vi "TP Buffer Search for Connection (No PGN).vi"(0 "Connecctions":T3[](array[typedef]), 5 "CAN frame":T1 {"payload" format="%x"; "timestamp" format="%<%.7X\n%x>T"; "type" items=["CAN Data"=0, "CAN Remote"=1, "CAN Bus Error"=2, "J1939 Data"=192, "Delay"=224, "Log Trigger"=225, "Start Trigger"=226]; "identifier" format="%x"}, 11 "error in (no error)":errorcluster) -> (4 "Connection Cluster Out":T3, 6 "CAN frame Out":T1 {"payload" format="%x"; "timestamp" format="%<%.7X\n%x>T"; "type" items=["CAN Data"=0, "CAN Remote"=1, "CAN Bus Error"=2, "J1939 Data"=192, "Delay"=224, "Log Trigger"=225, "Start Trigger"=226]; "identifier" format="%x"}, 8 "Found?":bool, 10 "Index":i32, 15 "error out":errorcluster)   [LabVIEW 2013, in "J1939.lvlib"]
uses:
  J1939.lvlib
  TP Buffer Connection Cluster.ctl
  <vilib>/xnet/xnet.llb/XNET Frame CAN.ctl
  <vilib>/xnet/xnet.llb/XNET Frame Type CAN.ctl
  Frame Conversion/Convert CAN Arb ID to J1939 ID.vi
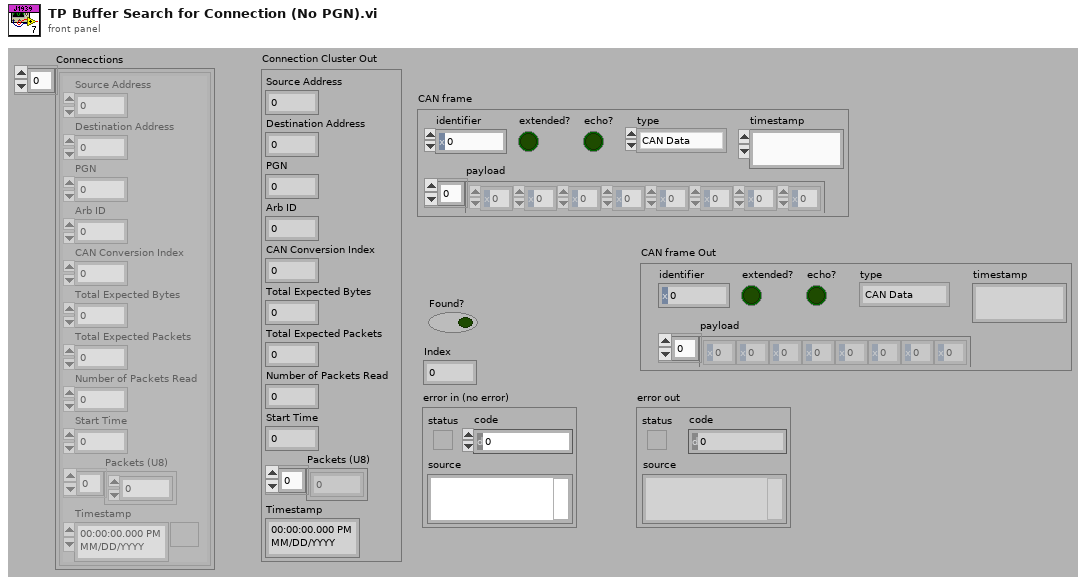
[diagram p1: front panel]
types:
  T1 = typedef "XNET Frame CAN.ctl" = cluster{"timestamp":timestamp, "payload":u8[], "identifier":u32, "type":T2, "extended?":bool, "echo?":bool}
  T2 = typedef "XNET Frame Type CAN.ctl" = u8
  T3 = typedef "J1939.lvlib/TP Buffer Connection Cluster.ctl" = cluster{"Source Address":u8, "Destination Address":u8, "PGN":u32, "Arb ID":u32, "CAN Conversion Index":u32, "Total Expected Bytes":u16, "Total Expected Packets":u8, "Number of Packets Read":u8, "Start Time":u32, "Packets (U8)":u8[], "Timestamp":timestamp}
  T4 = typedef "J1939.lvlib/PGN Fields Cluster.ctl" = cluster{"Reserved Bit":u8, "Data page":u8, "PDU Format":u8, "PDU Specific":u8}
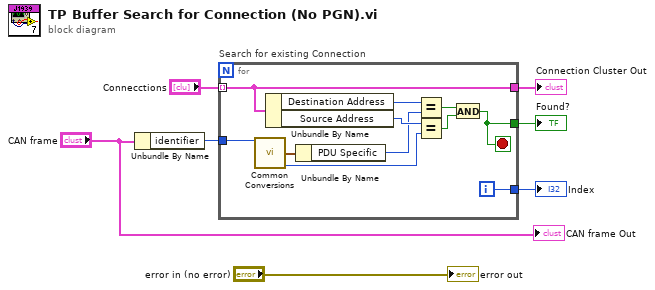
[diagram p0: block diagram]
diagram:
  n1 = Unbundle By Name("CAN frame") -> ("identifier"=w3:u32)
  n2 = for "Search for existing Connection" {
    tunnel: "Connecctions" -> [w9] mode=indexing
    tunnel: w3 -> [w16]
    tunnel: [w10] -> w7
    tunnel: [w9] -> w5
    tunnel: [w8] -> w4
    i -> [w8]
    stop <- w10 stop-if-true
    n3 = call-poly "Common Conversions.vi"("Arb ID"=w16) -> ("PGN Fields"=w17:T4, "Source Address"=w14:u8)  [unwired: 13 out]
    n4 = Unbundle By Name(w9) -> ("Destination Address"=w18:u8, "Source Address"=w15:u8)
    n5 = Unbundle By Name(w17) -> ("PDU Specific"=w13:u8)
    n6 = Equal?(x=w18, y=w13) -> (x = y?=w12:bool)
    n7 = Equal?(x=w15, y=w14) -> (x = y?=w11:bool)
    n8 = And(x=w12, y=w11) -> (x .and. y?=w10:bool)
  }
  "Found?" <- w7
  "Connection Cluster Out" <- w5
  "Index" <- w4
  "error out" <- "error in (no error)"
  "CAN frame Out" <- "CAN frame"
